vi "EventLog.New(error).vi"(7 "Source (All)":T1, 8 "error in":errorcluster, 10 "ErrData":T2) -> (0 "error out":errorcluster)   [LabVIEW 2016]
uses:
  CitTemplate/citTemplate.errData.ctl
  EventLog.EventSource.ctl
  Translator/Translator.Message.ctl
  EventLog.Event.ctl
  EventLog.EventLevel.ctl
  EventLog.Buffer.Action.ctl
  User/User.Global.vi
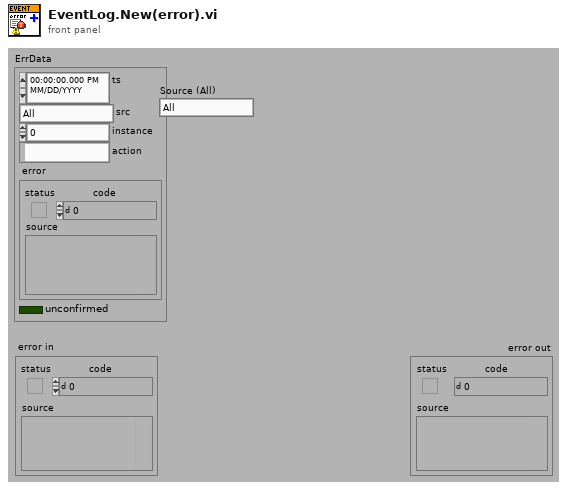
[diagram p1: front panel]
types:
  T1 = typedef "EventLog.EventSource.ctl" = enum16{"All", "Gui", "Ref", "File", "Arch", "Seq", "CPX", "DB", "Laser", "Scan.P", "Scan.O", "PLC"}
  T2 = typedef "citTemplate.errData.ctl" = cluster{"ts":timestamp, "src":T1, "instance":i32, "action":string, "error":errorcluster, "unconfirmed":bool}
  T3 = typedef "Translator.Message.ctl" = enum16{"-", "Event confirmed", "Log out", "Log in", "Shutdown", "Cancel", "Start", "Begin time", "End time", "Duration", "Service Mode", "Ignore Results", "Serial Format", "On", "Off", "OK", "NOK", "NOK %s", "Home", "Work", "Close", "Open", "In progress...", "Missing", "Empty", "Hardware failure", "Initial", "Default", "Total", "Out of range", "Free disk space is below 1GB - contact technician", "Error %d >> %s", "Error %d >> %s >> %s", "Msg %d >> %s", "Laser msg %d %s", "Laser cmd error %s %d", "Laser cmd failed %s", "Laser cmd warning %s", "Laser disconnected", "Laser status %s", "Laser already started", "Laser job unkonwn %s", "Laser job missing %s", "Laser job select failure %s", "Unable to start laser printing (%s)", "Unable to stop laser printing (%s)", "Laser marking aborted", "Laser marking timeout", "Unable to reset Laser Interlock (%s)", "Unable to trigger Laser. Laser not ready (%s)", "Laser job '%s' coordinates not configured", "Starting %s", "Quitting %s", "Configured", "Initializing", "Quitting", "Loading", "Loaded %d results", "Loaded %d events", "Running", "Stopped", "Summary", "Laser", "Do you want to continue?", "Do you want to delete the configuration?", "The configuration is being used by an order. Unable to delete!", "Press confirm button", "Station is not based. Do you want to exit?", "Station requires changeover. Do you want to run the test?", "Test options are not set as default. Do you want to continue?", "Formatting of WabcoNo is disabled. Do you want to continue?", "Product not detected. Do you want to continue?", "Product scan failed. Do you want to continue?", "Calibration", "Log out?", "System", "All", "IDLE", "Translating...%s", "Not found", "Alarm %s", "Run", "Skip", "Abort", "Repeat", "Please wait...", "Database disconnected", "Database disconnected - changeover disabled!", "Login to database successful", "Login to database failed: %d; %s", "Unable to check the product status of reference %d - database disconnected", "Unable to set the product status of reference %d - database disconnected", "Variant file backup %s", "Read variant (%s)", "Result", "Station armed!", "Station requires changeover!", "Select reference number...", "EMERGENCY BUTTON - press Control button", "EMERGENCY DOOR - press Control button", "Resetting Emergency...", "Unable to reset safety circuit - Emergency Button pressed", "Unable to reset safety circuit - Emergency Side Door open", "Station not based", "Station based", "Station not empty", "Station basing...", "No order", "Press Start to begin new order", "Scanning new order", "Order NOK. Correct or scan again", "Order OK. Press Accept", "Order ready", "Revolver incorrect", "Fork incorrect", "Revolver missing", "Revolver empty", "Container missing", "Offline results", "Offline statistics", "Updating statistics %.1f %%", "DMC Configurator", "Door open", "Close the front door", "Press start button", "Done. Open the front door", "Running...", "Running...%.1f %%", "Pause %s", "Pause %s. NOK container missing", "Pause %s. OK container missing", "Pause %s. Revolver empty", "Pause %s. Revolver missing", "Pause %s. Revolver incorrect", "Pause %s. Fork missing", "Pause %s. Fork incorrect", "Pause %s. Too many failures", "Pause %s. Unloading failure", "Pause %s. One slot is not working", "Pause %s. Part order is done. Empty OK container", "Pause %s. Unable to move product to slot", "Pause %s. Unable to move back product pusher", "Pause %s. Unable to lift product", "Pause %s. Unable to move back product lifter", "Pause %s. Unable to move product arm to Work", "Pause %s. Unable to move product arm to NOK", "Pause %s. Unable to move product arm to OK", "Pause %s. Unable to unsuck the NOK product", "Pause %s. Unable to drop the NOK product", "Pause %s. Product OK missing", "Pause %s. Unable to unsuck the OK product", "Pause %s. Unable to drop the OK product", "Stopping...", "File '%s' is missing", "File '%s' is broken", "File '%s' is running", "Log file started (%s)", "Log file ended (%s)", "Log file stopped (%s)", "Log file ignored (%s)", "Log file exported (%s)", "Log file export failed (%s)", "Wrong serial number in log file", "Wrong reference number in log file", "Test steps are missing", "%s = %.3f", "Process param '%s' not found in DB", "Process param '%s' wrong order", "Process param '%s' value %.3f out of limits (%.3f; %.3f)", "Step%d param '%s' not found in DB", "Step%d param '%s' wrong order", "Step%d param '%s' value %.3f out of limits (%.3f; %.3f)", "Step%d EV '%s' not found in DB", "Step%d EV '%s' wrong order", "\"%s\" not found in DB", "\"%s\" wrong order", "\"%s\" value %.3f out of limits (%.3f; %.3f)", "\"%s\" not found in software", "Process init (%s)", "Process started", "Process restarted", "Process run", "Process done", "Process done - remove OK container", "Process aborted", "Process aborted at work", "Process aborted at home", "Process error", "Process error at home", "Process error at work", "Process close", "Process pause", "Process continue", "Process door open", "Process door close", "Process pause at slot %s due to %s", "Select plate from the order to process", "Do you want to start the process?", "Do you want to continue the process?", "There is unfinished order. Do you want to put the new order?", "Product %s %d OK", "Product %s %d NOK", "Unable to unload the slot %s. Product missing in the slot", "Unable to unload the slot %s. Product already in the arm", "Unable to accept the product as OK. Product missing in slot %s", "Unable to accept the product as OK. Product could not drop into the container at slot %s", "Unable to accept the product as NOK. Product could not drop into the container at slot %s", "Scan failed. Error %s", "Scan failed. Scanner disconnected", "Scan failed. Wrong Wabco number %d, limit (%d,%d)", "Scan failed. Wrong serial number %d, limit (%d,%d)", "Scan failed. Wrong date %d, limit (%d,%d)", "Scan failed. Wrong product wabco number %d (expected %d)", "Scan failed. Wrong product serial number %d (expected > 0)", "Scan OK %s", "Scan failed. Unable to determine table position (%s)", "Scan failed. Timeout", "Tune failed. Scanner disconnected", "Tune failed. Timeout", "%s = %d", "%s = %d->%d", "Unable to set %s = %.2f - Air Pressure Inside off", "Unable to set digital output '%s' = %d", "Unable to activate air pressure inside - timeout", "Unable to activate air pressure inside - aborted", "Unable to switch on Air Main Valve - Air Pressure Inlet off", "Unable to switch on Air Main Valve - Door open", "Unable to switch off Air Main Valve - timeout", "Unable to switch off Air Main Valve - aborted", "Unable to rotate Table - timeout", "Unable to rotate Table - aborted", "Unable to rotate Table - Product Move not in Home position", "Unable to rotate Table - Air Pressure Inside off", "Unable to rotate Table - Product Lift A not in Home position", "Unable to rotate Table - Product Lift B not in Home position", "Unable to rotate Table - unlock before movement timeout", "Unable to rotate Table - lock after movement timeout", "Unable to move Table Lock to %s position - timeout", "Unable to move Table Lock to %s position - aborted", "Unable to move Table Lock to %s position - Air Pressure Inside off", "Unable to move Table Lock to %s position - Table not in position", "Unable to move Product Lift A to %s position - timeout", "Unable to move Product Lift B to %s position - timeout", "Unable to move Product Lift A to %s position - aborted", "Unable to move Product Lift B to %s position - aborted", "Unable to move Product Lift A to %s position - Air Pressure Inside off", "Unable to move Product Lift B to %s position - Air Pressure Inside off", "Unable to move Product Lift A to %s position - Table not locked", "Unable to move Product Lift B to %s position - Table not locked", "Unable to move Product Lift A to %s position - Product Arm not in Work position", "Unable to move Product Lift B to %s position - Product Arm not in Work position", "Unable to set Product Suction Gripper %s to %s - timeout", "Unable to set Product Suction Gripper %s to %s - aborted", "Unable to set Product Suction Gripper %s to %s - Air Pressure Inside off", "Unable to set Product Suction Gripper %s to %s - Table slot unkown", "Unable to move Product Arm to %s position - timeout", "Unable to move Product Arm to %s position - aborted", "Unable to move Product Arm to %s position - Air Pressure Inside off", "Unable to move Product Arm to %s position - Product Lift A not in Home position", "Unable to move Product Arm to %s position - Product Lift B not in Home position", "Unable to move Product to %s position - timeout", "Unable to move Product to %s position - aborted", "Unable to move Product to %s position - Air Pressure Inside off", "Unable to move Product to %s position - Table not in position"}
  T4 = typedef "EventLog.EventLevel.ctl" = enum8{"Debug", "Info", "Warning", "Error"}
  T5 = typedef "EventLog.Buffer.Action.ctl" = enum16{"init", "re-init", "clear", "set translator", "add", "get", "get unsaved"}
  T6 = typedef "EventLog.Event.ctl" = cluster{"ts":dbl, "lev":T4, "usr":i32, "src":T1, "msg":T3, "arg":variant[]}
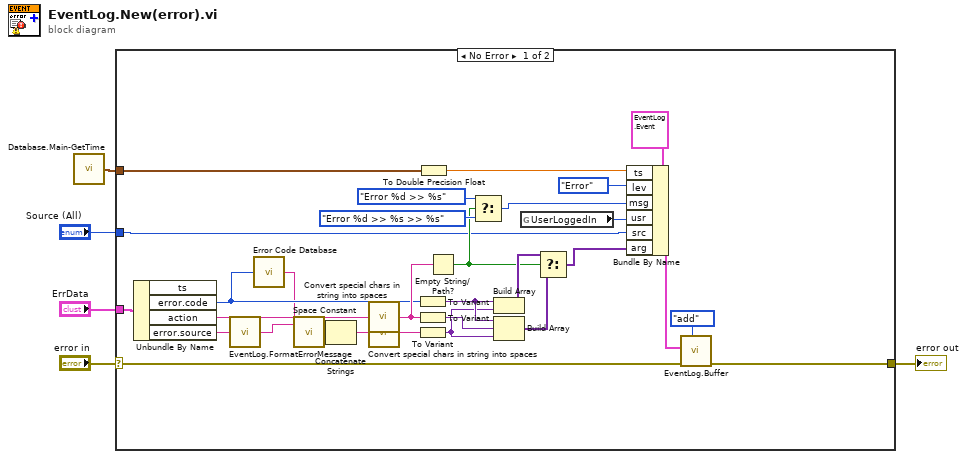
[diagram p0: block diagram]
diagram:
  n1 = call "Database.Main-GetTime.vi"() -> ("TS"=w1:timestamp)  [unwired: 1 in]
  n2 = case shown="No Error" "error in" {
    selector: "error in" -> [w14 w36]
    tunnel: [w13 w36] -> w5
    tunnel: "ErrData" -> [w31 _]
    tunnel: "Source (All)" -> [w17 _]
    tunnel: w1 -> [w6 _]
    frame No Error {
      n3 = Unbundle By Name(w31) -> ("error.code"=w12:i32, "action"=w30:string, "error.source"=w9:string)  [unwired: 1 out]
      n4 = call "EventLog.FormatErrorMessage.vi"("Error string in"=w9) -> ("Error string out"=w8:string)
      n5 = call <vilib>:"Error Code Database.vi"("Error Code"=w12) -> ("Error Text"=w7:string)
      n6 = call <vilib>:"Space Constant.vi"() -> ("String"=w10:string)
      n7 = Concatenate Strings(w8, w10, w7) -> (w11:string)
      n8 = call "Convert special chars in string into spaces.vi"("string with special characters"=w30) -> ("string with spaces"=w28:string)  [unwired: 2 in]
      n9 = call "Convert special chars in string into spaces.vi"("string with special characters"=w11) -> ("string with spaces"=w29:string)  [unwired: 2 in]
      n10 = To Variant(anything=w12) -> (Variant=w26:variant)
      n11 = To Variant(anything=w28) -> (Variant=w25:variant)
      n12 = To Variant(anything=w29) -> (Variant=w24:variant)
      n13 = To Double Precision Float(number=w6) -> (double precision float=w33:dbl)
      n14 = Empty String/Path?(string/path=w28) -> (empty?=w19:bool)
      n15 = Select(t=Translator.Message."Error %d >> %s" ("msg"), s=w19, f=Translator.Message."Error %d >> %s >> %s" ("msg")) -> (s? t:f=w18:T3)
      n16 = Build Array(w26, w24) -> (w27:variant[])
      n17 = Build Array(w26, w25, w24) -> (w23:variant[])
      n18 = global read "User.Global.vi" "UserLoggedIn"() -> (w32:i32)
      n19 = Select(t=w27, s=w19, f=w23) -> (s? t:f=w22:variant[])
      n20 = Bundle By Name(cluster=T6 {"ts"=0.0, "lev"=enum."Debug", "usr"=0, "src"=enum."All", "msg"=enum."Log out", "arg"=[]} ("Event in"), "ts"=w33, "lev"=EventLog.EventLevel."Error", "msg"=w18, "usr"=w32, "src"=w17, "arg"=w22) -> (w16:T6)
      n21 = call "EventLog.Buffer.vi"("action (get)"=EventLog.Buffer.Action."add" ("action (read)"), "error in"=w14, "Event in"=w16) -> ("error out"=w13:errorcluster)  [unwired: 5 in, 3 out]
    }
    frame Error {
    }
  }
  "error out" <- w5
